vi "TPNT_Args2DeviceInfo.vi"(9 "key":string, 10 "value":string, 11 "Device IN":T1={"device"="", "devupdate"=0.0, "next_update"=0, "devinterface"="", "TPs"=[], "Alarms"=TRUE, "monitor"=TRUE, "log sep"=""} {"TPs"."Log"."updaterate" format="%.2f"; "TPs"."Samples"."Values" format="%.2f"; "TPs"."Samples"."samples" min=1 step=1; "TPs"."Limits"."Nominal" format="%.2f"; "TPs"."Limits"."Upper" format="%.2f"; "TPs"."Limits"."Lower" format="%.2f"; "TPs"."update_rate" format="%.2f"; "devupdate" format="%.2f"}) -> (3 "Device OUT":T1={"device"="", "devupdate"=0.0, "next_update"=0, "devinterface"="", "TPs"=[], "Alarms"=TRUE, "monitor"=TRUE, "log sep"=""} {"TPs"."Log"."updaterate" format="%.2f"; "TPs"."Samples"."Values" format="%.2f"; "TPs"."Samples"."samples" min=1 step=1; "TPs"."Limits"."Nominal" format="%.2f"; "TPs"."Limits"."Upper" format="%.2f"; "TPs"."Limits"."Lower" format="%.2f"; "TPs"."update_rate" format="%.2f"; "devupdate" format="%.2f"})   [LabVIEW 2016]
uses:
  TPNT_DeviceTPs.ctl
  TPNT_TP.ctl
  TPNT_Limits.ctl
  TPNT_Samples.ctl
  TPNT_Log.ctl
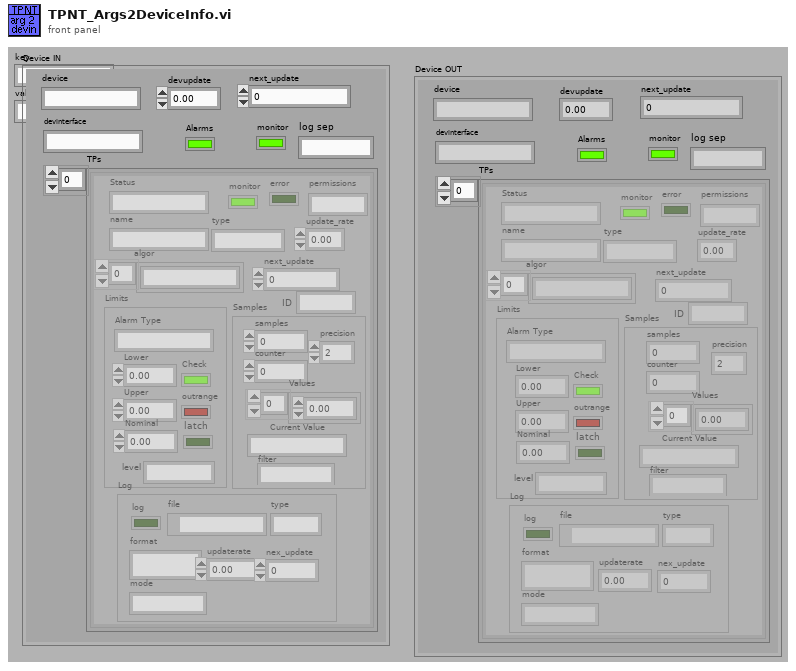
[diagram p1: front panel]
types:
  T1 = typedef "TPNT_DeviceTPs.ctl" = cluster{"device":string, "devupdate":dbl, "next_update":u32, "devinterface":string, "TPs":T2[], "Alarms":bool, "monitor":bool, "log sep":string}
  T2 = typedef "TPNT_TP.ctl" = cluster{"name":string, "type":string, "algor":string[], "update_rate":sgl, "Limits":T3, "Samples":T4, "next_update":u32, "Status":string, "monitor":bool, "error":bool, "Log":T5, "permissions":string, "ID":string}
  T3 = typedef "TPNT_Limits.ctl" = cluster{"Alarm Type":string, "Lower ":dbl, "Upper":dbl, "Nominal":dbl, "outrange":bool, "Check":bool, "latch":bool, "level":string}
  T4 = typedef "TPNT_Samples.ctl" = cluster{"samples":i32, "counter":i32, "Values":dbl[], "Current Value":string, "filter":string, "precision":u8}
  T5 = typedef "TPNT_Log.ctl" = cluster{"log":bool, "file":path, "type":string, "format":string, "updaterate":dbl, "nex_update":u32, "mode":string}
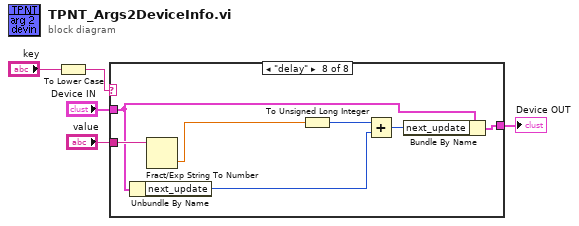
[diagram p0: block diagram]
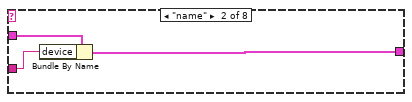
[diagram p3: hidden frame]
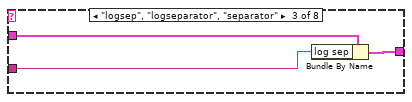
[diagram p4: hidden frame]
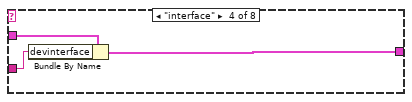
[diagram p5: hidden frame]
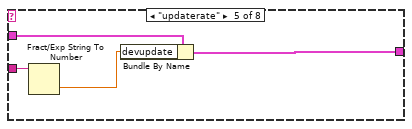
[diagram p6: hidden frame]
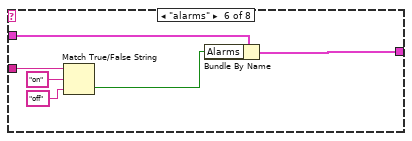
[diagram p7: hidden frame]
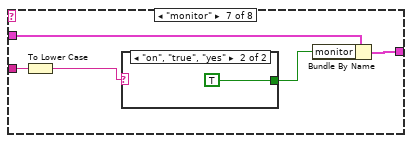
[diagram p8: hidden frame]
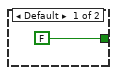
[diagram p9: hidden frame]
diagram:
  n1 = To Lower Case(string="key") -> (all lower case string=w4:string)
  n2 = case shown="\"delay\"" w4 {
    tunnel: "value" -> [_ w9 w10 w15 w19 w23 w27 w39]
    tunnel: "Device IN" -> [w6 w8 w12 w14 w17 w25 w30 w37]
    tunnel: [w6 w7 w11 w13 w16 w24 w29 w38] -> w1
    frame Default {
    }
    frame "name" {
      n3 = Bundle By Name(cluster=w8, "device"=w9) -> (w7:T1)
    }
    frame "logsep", "logseparator", "separator" {
      n4 = Bundle By Name(cluster=w12, "log sep"=w10) -> (w11:T1)
    }
    frame "interface" {
      n5 = Bundle By Name(cluster=w14, "devinterface"=w15) -> (w13:T1)
    }
    frame "updaterate" {
      n6 = Fract/Exp String To Number(string=w19) -> (number=w18:dbl)  [unwired: 4 out]
      n7 = Bundle By Name(cluster=w17, "devupdate"=w18) -> (w16:T1)
    }
    frame "alarms" {
      n8 = Match True/False String(2:"off" ("false string"), 3:"on" ("true string"), 4:w23) -> (0:w20:bool)  [unwired: 1 out]
      n9 = Bundle By Name(cluster=w25, "Alarms"=w20) -> (w24:T1)
    }
    frame "monitor" {
      n10 = To Lower Case(string=w27) -> (all lower case string=w26:string)
      n11 = case shown="\"on\", \"true\", \"yes\"" w26 {
        tunnel: [FALSE TRUE] -> w28
        frame Default {
        }
        frame "on", "true", "yes" {
        }
      }
      n12 = Bundle By Name(cluster=w30, "monitor"=w28) -> (w29:T1)
    }
    frame "delay" {
      n13 = Unbundle By Name(w37) -> ("next_update"=w35:u32)
      n14 = Fract/Exp String To Number(string=w39) -> (number=w33:dbl)  [unwired: 4 out]
      n15 = To Unsigned Long Integer(number=w33) -> (unsigned 32bit integer=w36:u32)
      n16 = Add(x=w36, y=w35) -> (x+y=w34:u32)
      n17 = Bundle By Name(cluster=w37, "next_update"=w34) -> (w38:T1)
    }
  }
  "Device OUT" <- w1
